vi "Destroy Discovery.vi"(8 "error in (no error)":errorcluster, 11 "CIFPluginManager in":refnum<class "CIFPluginManager.lvclass">) -> (0 "error out":errorcluster, 3 "CIFPluginManager out":refnum<class "CIFPluginManager.lvclass">)   [LabVIEW 2021, in "CIFPluginManager.lvclass"]
uses:
  CIFPluginManager.lvclass
  CIFPluginManager.lvclass/CIFPluginManager.ctl
  typedef/Trigger Discovery User Event.ctl
  CIFCore/Common/Typedef/Version.ctl
  CIFCore/Common/CIFCoreCommon.lvlib
  typedef/Plugin Metadata.ctl
  typedef/Discovered Plugin.ctl
  typedef/Discovery User Event.ctl
  typedef/Discovery Events.ctl
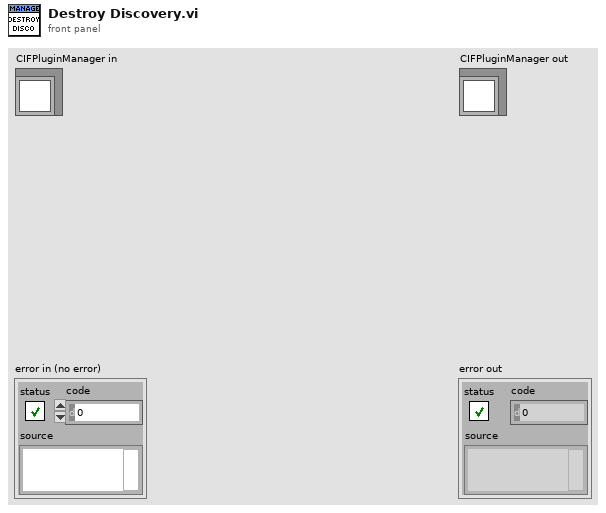
[diagram p1: front panel]
types:
  T1 = typedef "CIFPluginManager.lvclass/Discovery Events.ctl" = cluster{"Trigger Discovery":T2, "Discovery":T3, "Shutdown":refnum<user-event>}
  T2 = typedef "CIFPluginManager.lvclass/Trigger Discovery User Event.ctl" = refnum<user-event>
  T3 = typedef "CIFPluginManager.lvclass/Discovery User Event.ctl" = refnum<user-event>
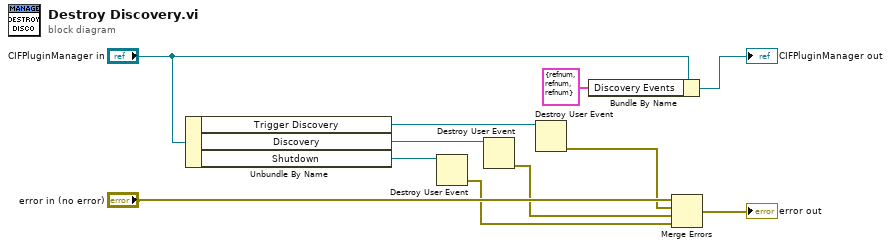
[diagram p0: block diagram]
diagram:
  n1 = Unbundle By Name("CIFPluginManager in") -> ("Trigger Discovery"=w6:T2, "Discovery"=w7:T3, "Shutdown"=w8:refnum<user-event>)
  n2 = Destroy User Event(user event=w8) -> (error out=w2:errorcluster)  [unwired: 1 in]
  n3 = Destroy User Event(user event=w7) -> (error out=w3:errorcluster)  [unwired: 1 in]
  n4 = Destroy User Event(user event=w6) -> (error out=w4:errorcluster)  [unwired: 1 in]
  n5 = Bundle By Name(cluster="CIFPluginManager in", "Discovery Events"=T1 {"Trigger Discovery"=refnum, "Discovery"=refnum, "Shutdown"=refnum}) -> (→"CIFPluginManager out":refnum<class "CIFPluginManager.lvclass">)
  n6 = Merge Errors("error in (no error)", w4, w3, w2) -> (→"error out":errorcluster)
